vi "optogeneticsExecuteIntensityScan.vi"() -> ()   [LabVIEW 2017]
uses:
  globalDevices.vi
  globalUtilities.vi
panel:
  out "elapsed time (s)":dbl
  out "pharosFire":bool
  out "currentRepRateDivider":i32
  out "currentNPulses":i32
  in  "executeStep":bool
  in  "stimulus duration (s)":dbl=1.0
  in  "repRateDivider":i32[](array[numeric])=[1]
  out "nPulses":i32[](array[numeric])
  # "SCAN IN INTENSITY WITH FIXED PULSE TRAIN DURATION\nEnable external control in pharosControl.\nUse the appropriate software for spatial targeting. This VI only deals with the laser pulses."
  # "EXECUTE STEP AND FIRE LASER PULSES"
  # "DIAGNOSTICS"
  # "SET"
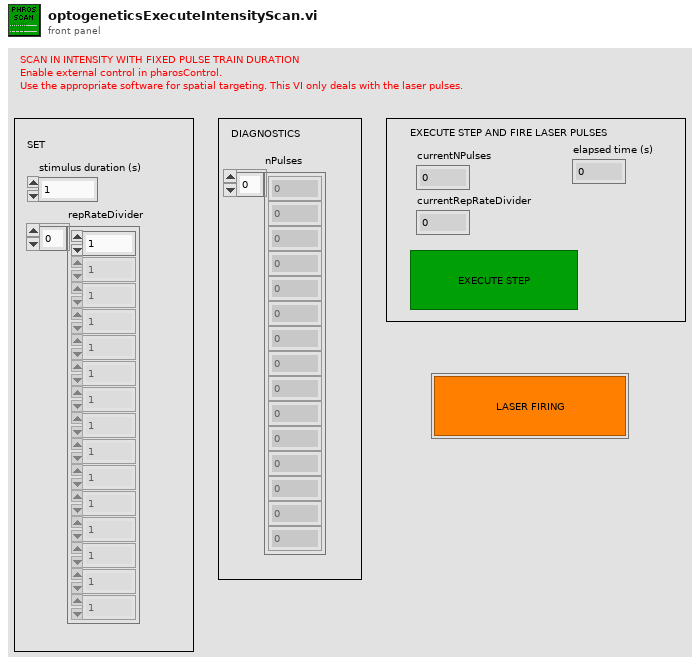
[diagram p1: front panel]
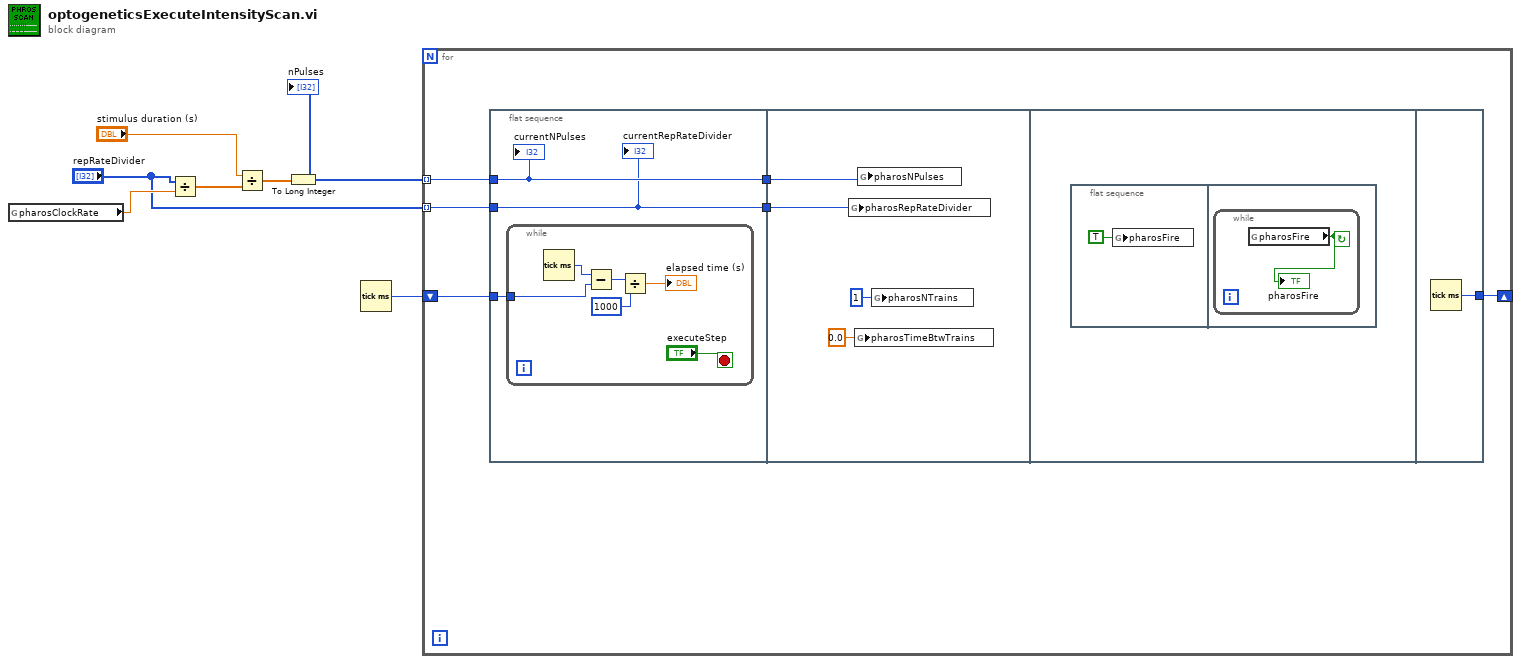
[diagram p0: block diagram]
diagram:
  n1 = global read "globalDevices.vi" "pharosClockRate"() -> (w7:dbl)
  n2 = Divide(x="repRateDivider", y=w7) -> (x/y=w5:dbl[])
  n3 = Divide(x="stimulus duration (s)", y=w5) -> (x/y=w4:dbl[])
  n4 = To Long Integer(number=w4) -> (32bit integer=w3:i32[])
  "nPulses" <- w3
  n5 = Tick Count (ms)() -> (millisecond timer value=w1:u32)
  n6 = for {
    tunnel: w3 -> [w12] mode=indexing
    tunnel: "repRateDivider" -> [w10] mode=indexing
    shift-right: [w8] -> _
    shift-left: w1 -> [w9]
    n7 = flat-sequence {
      tunnel: [w16] -> w13
      tunnel: w12 -> [w16]
      tunnel: [w15] -> w11
      tunnel: w10 -> [w15]
      tunnel: w9 -> [w14]
      tunnel: w13 -> [w24]
      tunnel: w11 -> [w23]
      tunnel: [w29] -> w8
      frame #0 {
        n8 = while {
          tunnel: w14 -> [w20]
          stop <- "executeStep" stop-if-true
          n9 = Tick Count (ms)() -> (millisecond timer value=w21:u32)
          n10 = Subtract(x=w21, y=w20) -> (x-y=w19:u32)
          n11 = Divide(x=w19, y=u32 1000) -> (x/y=→"elapsed time (s)":dbl)
        }
        "currentNPulses" <- w16
        "currentRepRateDivider" <- w15
      }
      frame #1 {
        n12 = global write "globalUtilities.vi" "pharosRepRateDivider"(w23) -> ()
        n13 = global write "globalUtilities.vi" "pharosTimeBtwTrains"(0.0 ("pharosTimeBtwTrains")) -> ()
        n14 = global write "globalUtilities.vi" "pharosNPulses"(w24) -> ()
        n15 = global write "globalUtilities.vi" "pharosNTrains"(1 ("pharosNTrains")) -> ()
      }
      frame #2 {
        n16 = flat-sequence {
          frame #0 {
            n17 = global write "globalUtilities.vi" "pharosFire"(TRUE ("pharosFire")) -> ()
          }
          frame #1 {
            n18 = while {
              stop <- w28 continue-if-true
              n19 = global read "globalUtilities.vi" "pharosFire"() -> (w28:bool)
              "pharosFire" <- w28
            }
          }
        }
      }
      frame #3 {
        n20 = Tick Count (ms)() -> (millisecond timer value=w29:u32)
      }
    }
  }
